vi "Error Bar Constructor.vi"(5 "error b vector":dbl[](array[numeric]), 7 "error a vector":dbl[](array[numeric]), 8 "error in (no error)":errorcluster, 9 "y vector":dbl[](array[numeric]), 10 "x vector":dbl[](array[numeric]), 11 "2D Error Bar Datatype.lvclass in":refnum<class "2D Error Bar Datatype.lvclass">) -> (0 "error out":errorcluster, 3 "2D Error Bar Datatype.lvclass out":refnum<class "2D Error Bar Datatype.lvclass">)   [LabVIEW 2017, in "2D Error Bar Datatype.lvclass"]
uses:
  <vilib>/Math Plots/2D Math Plots/2D Error Bar/2D Error Bar Datatype/2D Error Bar Datatype.lvclass
  <vilib>/Math Plots/2D Math Plots/2D Error Bar/2D Error Bar Datatype/2D Error Bar Datatype.lvclass/2D Error Bar Datatype.ctl
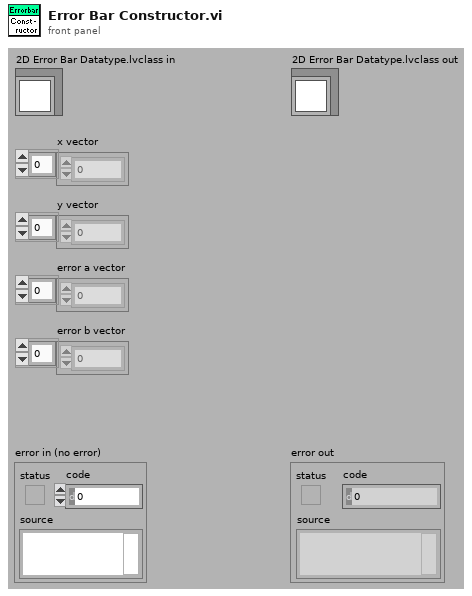
[diagram p1: front panel]
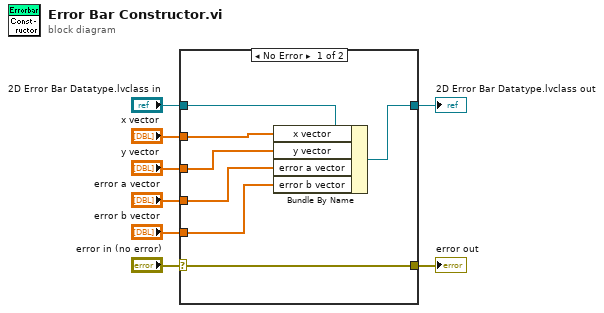
[diagram p0: block diagram]
diagram:
  n1 = case shown="No Error" "error in (no error)" {
    selector: "error in (no error)" -> [w15 w17]
    tunnel: [w15 w17] -> w4
    tunnel: "x vector" -> [w13 _]
    tunnel: "y vector" -> [w12 _]
    tunnel: "2D Error Bar Datatype.lvclass in" -> [w14 w16]
    tunnel: [w11 w16] -> w8
    tunnel: "error a vector" -> [w10 _]
    tunnel: "error b vector" -> [w9 _]
    frame No Error {
      n2 = Bundle By Name(cluster=w14, "x vector"=w13, "y vector"=w12, "error a vector"=w10, "error b vector"=w9) -> (w11:refnum<class "2D Error Bar Datatype.lvclass">)
    }
    frame Error {
    }
  }
  "error out" <- w4
  "2D Error Bar Datatype.lvclass out" <- w8
